vi "dvr.vi"(11 "Error In":errorcluster, 13 "DVR Operation":T1) -> (4 "DVR Ref":refnum<data-value>, 15 "Error Out":errorcluster)   [LabVIEW 2020, in "I2C Controller.lvlib" / "Protocols.lvclass"]
uses:
  Protocols.lvclass
  Typedef's/DVR Operations.ctl
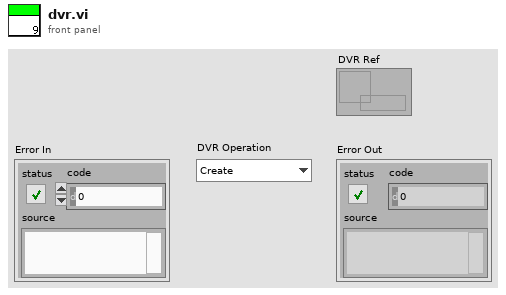
[diagram p1: front panel]
types:
  T1 = typedef "I2C Controller.lvlib/Protocols.lvclass/DVR Operations.ctl" = enum16{"Create", "Destroy"}
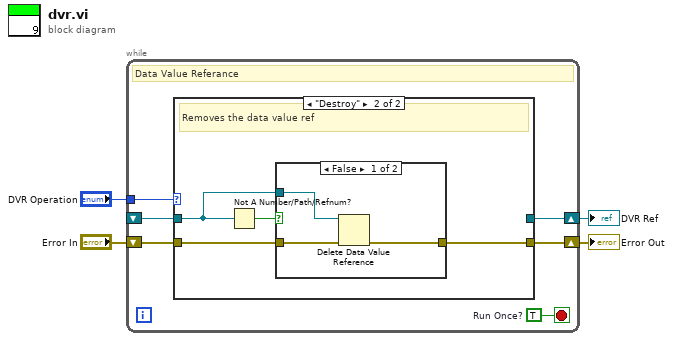
[diagram p0: block diagram]
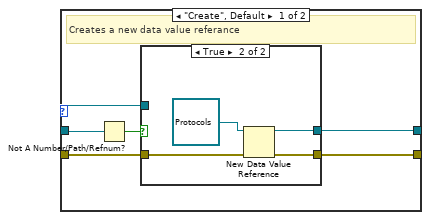
[diagram p2: hidden frame]
diagram:
  n1 = while {
    tunnel: "DVR Operation" -> [w9]
    shift-right: [w7] -> w2
    shift-left: "Error In" -> [w8]
    shift-right: [w6] -> w1
    shift-left: _ -> [w5]
    stop <- w10 stop-if-true
    w10 = TRUE  # Run Once?
    # "Data Value Referance"
    n2 = case shown="\"Destroy\"" w9 {
      tunnel: w8 -> [w15 w25]
      tunnel: [w14 w24] -> w7
      tunnel: [w13 _] -> w6
      tunnel: w5 -> [w11 w22]
      frame "Create", Default {
        # "Creates a new data value referance"
        n3 = Not A Number/Path/Refnum?(number/path/refnum=w11) -> (NaN/Path/Refnum?=w12:bool)
        n4 = case shown="True" w12 {
          tunnel: w15 -> [w16 w21]
          tunnel: [w16 w20] -> w14
          tunnel: [w17 w18] -> w13
          tunnel: w11 -> [w17 _]
          frame False {
          }
          frame True {
            n5 = New Data Value Reference(data value=refnum<class "Protocols.lvclass"> refnum ("I2C Controller.lvlib:Protocols.lvclass"), error in=w21) -> (data value reference=w18:refnum<data-value>, error out=w20:errorcluster)
          }
        }
      }
      frame "Destroy" {
        # "Removes the data value ref"
        n6 = Not A Number/Path/Refnum?(number/path/refnum=w22) -> (NaN/Path/Refnum?=w23:bool)
        n7 = case shown="False" w23 {
          tunnel: w25 -> [w28 w29]
          tunnel: [w27 w29] -> w24
          tunnel: w22 -> [w26 _]
          frame False {
            n8 = Delete Data Value Reference(data value reference=w26, error in=w28) -> (error out=w27:errorcluster)  [unwired: 1 out]
          }
          frame True {
          }
        }
      }
    }
  }
  "Error Out" <- w2
  "DVR Ref" <- w1
